vi "Moving Chuck Test.vi"() -> ()   [LabVIEW 2017]
panel:
  out "Status":string
  in  "Stop":bool
  in  "Move":bool
  out "Error Out":errorcluster
  in  "Error In":errorcluster
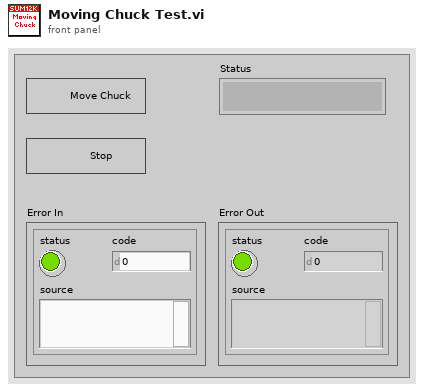
[diagram p1: front panel]
types:
  T1 = typedef "RegistrationNumber.ctl" = i32
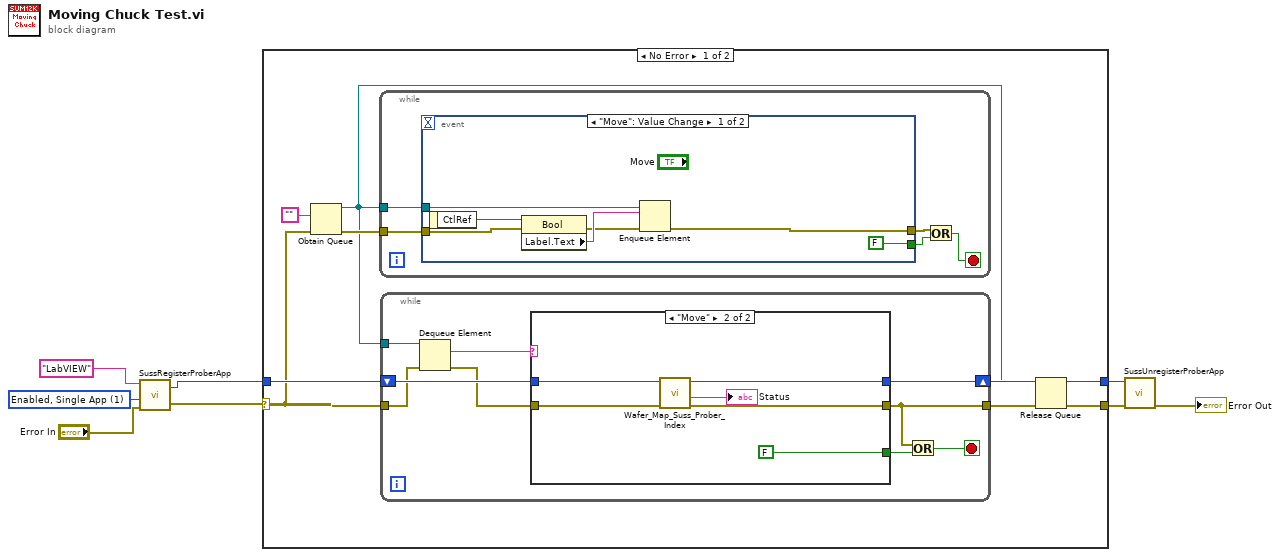
[diagram p0: block diagram]
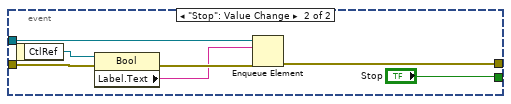
[diagram p2: hidden frame]
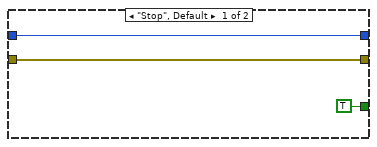
[diagram p3: hidden frame]
diagram:
  w8 = 1 items=["Disabled, Multiple App", "Enabled, Single App", "Disabled, Single App"] ("Flag")
  n1 = call "SussRegisterProberApp.vi"("error in (no error)"="Error In", "Flag"=w8, "Groupname"="LabVIEW") -> ("error out"=w2:errorcluster, "RegistrationNumber"=w1:T1)  [unwired: 1 in]
  n2 = case shown="No Error" w2 {
    selector: w2 -> [w13 w55]
    tunnel: w1 -> [w16 w54]
    tunnel: [w15 w54] -> w5
    tunnel: [w11 w55] -> w4
    frame No Error {
      n3 = Obtain Queue(element data type="", error in (no error)=w13) -> (queue out=w10:refnum<queue>, error out=w14:errorcluster)  [unwired: 3 in, 1 out]
      n4 = while {
        tunnel: w14 -> [w21]
        tunnel: w10 -> [w20]
        stop <- w19 stop-if-true
        n5 = event shown="[0] \"Move\": Value Change" {
          selector: _ -> [_ _]
          dyn-events: _ -> [_ _]
          timeout: _ -> [_ _]
          tunnel: w21 -> [w27 w33]
          tunnel: w20 -> [w24 w31]
          tunnel: [w23 w29] -> w18
          tunnel: [FALSE "Stop"] -> w17
          event "Move": Value Change {
            n6 = event-data() -> ("CtlRef"=w28:refnum<vi>)  [unwired: 1 in]
            n7 = property class="Bool"(reference=w28, error in=w27) -> (error out=w25:errorcluster, "Label.Text"=w26:string)  [unwired: 1 out]
            n8 = Enqueue Element(queue=w24, element=w26, error in (no error)=w25) -> (error out=w23:errorcluster)  [unwired: 1 in, 2 out]
          }
          event "Stop": Value Change {
            n9 = event-data() -> ("CtlRef"=w34:refnum<vi>)  [unwired: 1 in]
            n10 = property class="Bool"(reference=w34, error in=w33) -> (error out=w32:errorcluster, "Label.Text"=w30:string)  [unwired: 1 out]
            n11 = Enqueue Element(queue=w31, element=w30, error in (no error)=w32) -> (error out=w29:errorcluster)  [unwired: 1 in, 2 out]
          }
        }
        n12 = Or(x=w18, y=w17) -> (x .or. y?=w19:bool)
      }
      n13 = while {
        shift-right: [w43] -> w15
        shift-left: w16 -> [w44]
        tunnel: w10 -> [w42]
        tunnel: w13 -> [w41]
        tunnel: [w37] -> w12
        stop <- w38 stop-if-true
        n14 = Dequeue Element(queue=w42, error in (no error)=w41) -> (element=w40:string, error out=w39:errorcluster)  [unwired: 1 in, 2 out]
        n15 = case shown="\"Move\"" w40 {
          tunnel: w39 -> [w47 w53]
          tunnel: w44 -> [w46 w52]
          tunnel: [w46 w51] -> w43
          tunnel: [w47 w50] -> w37
          tunnel: [TRUE FALSE] -> w36
          frame "Stop", Default {
          }
          frame "Move" {
            n16 = call "Wafer_Map_Suss_Prober_Index.vi"("error in (no error)"=w53, "RegistrationNumber"=w52) -> ("error out"=w50:errorcluster, "ResponseString 2"=→"Status":string, "RegistrationNumber out"=w51:T1)  [unwired: 6 in, 1 out]
          }
        }
        n17 = Or(x=w37, y=w36) -> (x .or. y?=w38:bool)
      }
      n18 = Release Queue(queue=w10, error in (no error)=w12) -> (error out=w11:errorcluster)  [unwired: 1 in, 2 out]
    }
    frame Error {
    }
  }
  n19 = call "SussUnregisterProberApp.vi"("error in"=w4, "RegistrationNumber"=w5) -> ("error out"=→"Error Out":errorcluster)  [unwired: 9 in]
